vi "BRig_RT__Case_Exp__State_initBlock.vi"(0 "input_dataCurrent":u16[](array[numeric]), 3 "input_dataExp":u16[](array[numeric]), 4 "input_dataBlock":u16[][](array[numeric]), 5 "input_dataTrial":u16[][](array[numeric])) -> (6 "output_iSpout":u16, 7 "output_speaker_amp_R":u16, 8 "output_iBlock":u16, 9 "output_speaker_freq_R":u8, 10 "output_BUR_target":u16, 11 "output_speaker_amp_L":u16, 12 "output_TpB_target":u16, 13 "output_speaker_freq_L":u8, 14 "output_dataCurrent":u16[](array[numeric]), 18 "output_dataBlock":u16[][](array[numeric]), 19 "output_dataTrial":u16[][](array[numeric]))   [LabVIEW 2014]
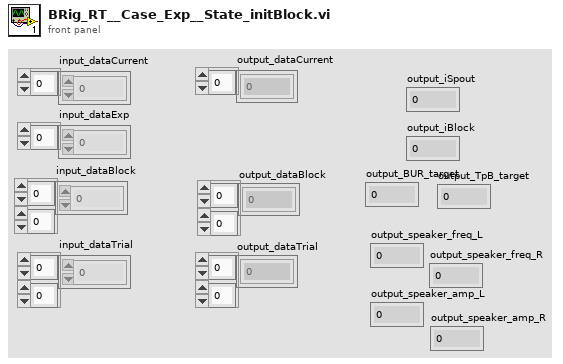
[diagram p1: front panel]
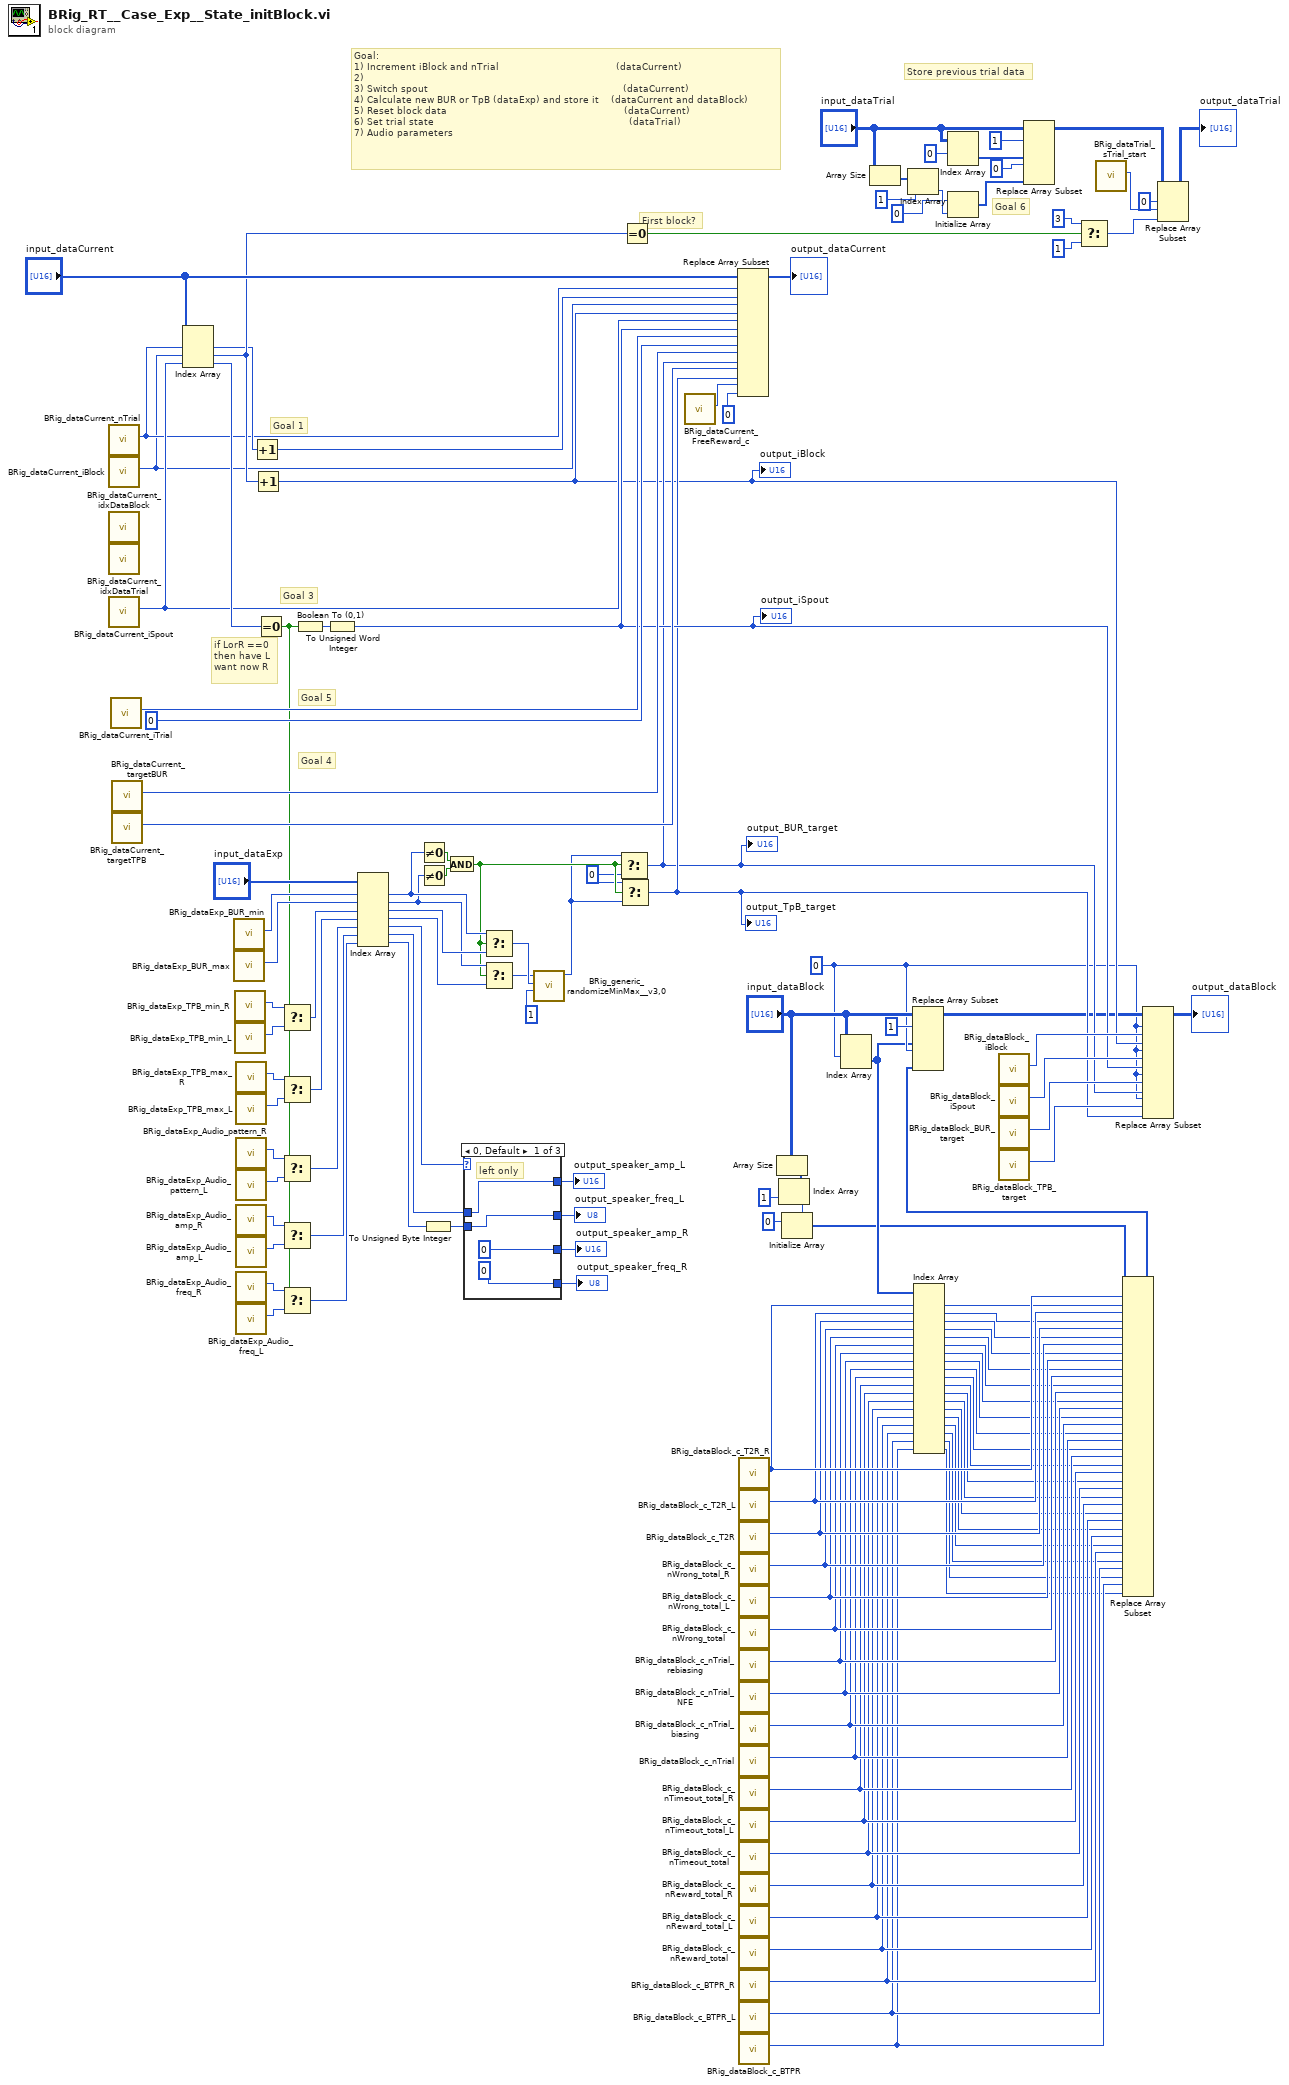
[diagram p0: block diagram]
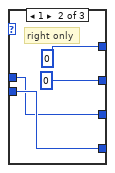
[diagram p2: hidden frame]
diagram:
  w43 = 0 ("disabled index (row)")
  w110 = u16 0 ("f")
  # "Store previous trial data"
  # "if LorR ==0\nthen have L\nwant now R"
  # "First block?"
  # "Goal 6"
  # "Goal 4"
  # "Goal 5"
  # "Goal 3"
  # "Goal 1"
  # "Goal:\n1) Increment iBlock and nTrial                                       (dataCurrent)\n2) \n3) Switch spout                                                                 (dataCurrent)\n4) Calculate new BUR or TpB (dataExp) and store it    (dataCurrent and dataBlock)\n5) Reset block data                                                           (dataCurrent)\n6) Set trial state                                                                 (dataTrial)\n7) Audio parameters"
  n1 = call "BRig_dataCurrent_nTrial.vi"() -> ("output_nTrial"=w65:i32)  [unwired: 11 in]
  n2 = call "BRig_dataCurrent_iBlock.vi"() -> ("output_iBlock"=w63:i32)  [unwired: 11 in]
  n3 = call "BRig_dataCurrent_idxDataBlock.vi"() -> ()  [unwired: 11 in, 1 out]
  n4 = call "BRig_dataCurrent_idxDataTrial.vi"() -> ()  [unwired: 11 in, 1 out]
  n5 = call "BRig_dataCurrent_iSpout.vi"() -> ("output_iSpout"=w93:i32)  [unwired: 11 in]
  n6 = call "BRig_dataCurrent_iTrial.vi"() -> ("output_iTrial"=w95:i32)  [unwired: 11 in]
  n7 = call "BRig_dataCurrent_targetBUR.vi"() -> ("output_targetBUR"=w97:i32)  [unwired: 11 in]
  n8 = call "BRig_dataCurrent_targetTPB.vi"() -> ("output_targetTPB"=w98:i32)  [unwired: 11 in]
  n9 = Index Array(array="input_dataCurrent", index #1=w65, index #2=w63, index #3=w93) -> (element #1=w92:u16, element #2=w104:u16, element #3=w129:u16)
  n10 = call "BRig_dataExp_BUR_min.vi"() -> ("output_BUR_min"=w127:i32)  [unwired: 11 in]
  n11 = call "BRig_dataExp_BUR_max.vi"() -> ("output_BUR_max"=w126:i32)  [unwired: 11 in]
  n12 = call "BRig_dataExp_TPB_min_R.vi"() -> ("output_TPB_min_R"=w122:i32)  [unwired: 11 in]
  n13 = call "BRig_dataExp_TPB_min_L.vi"() -> ("output_TPB_min_L"=w121:i32)  [unwired: 11 in]
  n14 = call "BRig_dataExp_TPB_max_R.vi"() -> ("output_TPB_max_R"=w68:i32)  [unwired: 11 in]
  n15 = call "BRig_dataExp_TPB_max_L.vi"() -> ("output_TPB_max_L"=w67:i32)  [unwired: 11 in]
  n16 = call "BRig_dataExp_Audio_pattern_R.vi"() -> ("output_Audio_sp__R"=w90:i32)  [unwired: 11 in]
  n17 = call "BRig_dataExp_Audio_pattern_L.vi"() -> ("output_Audio_sp__L"=w89:i32)  [unwired: 11 in]
  n18 = call "BRig_dataExp_Audio_amp_R.vi"() -> ("output_Audio_amp__R"=w88:i32)  [unwired: 11 in]
  n19 = call "BRig_dataExp_Audio_amp_L.vi"() -> ("output_Audio_amp__L"=w87:i32)  [unwired: 11 in]
  n20 = call "BRig_dataExp_Audio_freq_R.vi"() -> ("output_Audio_freq__R"=w86:i32)  [unwired: 11 in]
  n21 = call "BRig_dataExp_Audio_freq_L.vi"() -> ("output_Audio_freq__L"=w85:i32)  [unwired: 11 in]
  n22 = Increment(x=w92) -> (x+1=w64:u16)
  n23 = Increment(x=w104) -> (x+1=w62:u16)
  "output_iBlock" <- w62
  n24 = Equal To 0?(x=w129) -> (x = 0?=w91:bool)
  n25 = Select(t=w122, s=w91, f=w121) -> (s? t:f=w120:i32)
  n26 = Select(t=w68, s=w91, f=w67) -> (s? t:f=w119:i32)
  n27 = Select(t=w90, s=w91, f=w89) -> (s? t:f=w84:i32)
  n28 = Select(t=w88, s=w91, f=w87) -> (s? t:f=w83:i32)
  n29 = Select(t=w86, s=w91, f=w85) -> (s? t:f=w82:i32)
  n30 = Boolean To (0,1)(Boolean=w91) -> (0, 1=w130:i16)
  n31 = To Unsigned Word Integer(number=w130) -> (unsigned 16bit integer=w94:u16)
  "output_iSpout" <- w94
  n32 = Index Array(array="input_dataExp", index #1=w127, index #2=w126, index #3=w120, index #4=w119, index #5=w84, index #6=w83, index #7=w82) -> (element #1=w118:u16, element #2=w116:u16, element #3=w117:u16, element #4=w115:u16, element #5=w81:u16, element #6=w80:u16, element #7=w79:u16)
  n33 = Not Equal To 0?(x=w118) -> (x != 0?=w124:bool)
  n34 = Not Equal To 0?(x=w116) -> (x != 0?=w125:bool)
  n35 = To Unsigned Byte Integer(number=w79) -> (unsigned 8bit integer=w78:u8)
  n36 = And(x=w124, y=w125) -> (x .and. y?=w111:bool)
  n37 = case shown="0, Default" w81 {
    tunnel: w80 -> [w135 w138 w140]
    tunnel: w78 -> [w134 w139 w141]
    tunnel: [w135 u16 0 ("Numeric") w140] -> w77
    tunnel: [w134 u8 0 w141] -> w76
    tunnel: [u8 0 w139 w141] -> w75
    tunnel: [u16 0 ("Numeric") w138 w140] -> w74
    frame 0, Default {
      # "left only"
    }
    frame 1 {
      # "right only"
    }
    frame 2 {
      # "left and right"
    }
  }
  "output_speaker_amp_L" <- w77
  "output_speaker_freq_L" <- w76
  "output_speaker_amp_R" <- w74
  "output_speaker_freq_R" <- w75
  n38 = Select(t=w118, s=w111, f=w117) -> (s? t:f=w113:u16)
  n39 = Select(t=w116, s=w111, f=w115) -> (s? t:f=w112:u16)
  n40 = call "BRig_generic_randomizeMinMax__v3,0.vi"("Input_Increment"=u16 1, "Input_Min"=w113, "Input_Max"=w112) -> ("Output"=w109:u16)  [unwired: 8 in]
  n41 = Select(t=w109, s=w111, f=w110) -> (s? t:f=w72:u16)
  "output_BUR_target" <- w72
  n42 = Select(t=w110, s=w111, f=w109) -> (s? t:f=w73:u16)
  "output_TpB_target" <- w73
  n43 = Equal To 0?(x=w104) -> (x = 0?=w71:bool)
  n44 = call "BRig_dataCurrent_FreeReward_c.vi"() -> ("output_FreeReward_c"=w70:i32)  [unwired: 11 in]
  n45 = Replace Array Subset(array="input_dataCurrent", new element #1=w64, index #1=w65, new element #2=w62, index #2=w63, new element #3=w94, index #3=w93, new element #4=u16 0 ("new element/subarray"), index #4=w95, new element #5=w72, index #5=w97, new element #6=w73, index #6=w98, new element #7=u16 0 ("new element/subarray"), index #7=w70) -> (→"output_dataCurrent":u16[])
  n46 = call "BRig_dataBlock_c_T2R_R.vi"() -> ("output_c_T2R_R"=w38:i32)  [unwired: 11 in]
  n47 = call "BRig_dataBlock_c_T2R_L.vi"() -> ("output_c_T2R_L"=w37:i32)  [unwired: 11 in]
  n48 = call "BRig_dataBlock_c_T2R.vi"() -> ("output_c_T2R"=w36:i32)  [unwired: 11 in]
  n49 = call "BRig_dataBlock_c_nWrong_total_R.vi"() -> ("output_c_nWrong_total_R"=w35:i32)  [unwired: 11 in]
  n50 = call "BRig_dataBlock_c_nWrong_total_L.vi"() -> ("output_c_nWrong_total_L"=w34:i32)  [unwired: 11 in]
  n51 = call "BRig_dataBlock_c_nWrong_total.vi"() -> ("output_c_nWrong_total"=w33:i32)  [unwired: 11 in]
  n52 = call "BRig_dataBlock_c_nTrial_rebiasing.vi"() -> ("output_c_nTrial_rebiasing"=w32:i32)  [unwired: 11 in]
  n53 = call "BRig_dataBlock_c_nTrial_NFE.vi"() -> ("output_c_nTrial_NFE"=w31:i32)  [unwired: 11 in]
  n54 = call "BRig_dataBlock_c_nTrial_biasing.vi"() -> ("output_c_nTrial_biasing"=w30:i32)  [unwired: 11 in]
  n55 = call "BRig_dataBlock_c_nTrial.vi"() -> ("output_c_nTrial"=w29:i32)  [unwired: 11 in]
  n56 = call "BRig_dataBlock_c_nTimeout_total_R.vi"() -> ("output_c_nTimeout_total_R"=w28:i32)  [unwired: 11 in]
  n57 = call "BRig_dataBlock_c_nTimeout_total_L.vi"() -> ("output_c_nTimeout_total_L"=w27:i32)  [unwired: 11 in]
  n58 = call "BRig_dataBlock_c_nTimeout_total.vi"() -> ("output_c_nTimeout_total"=w26:i32)  [unwired: 11 in]
  n59 = call "BRig_dataBlock_c_nReward_total_R.vi"() -> ("output_nReward_total_R"=w25:i32)  [unwired: 11 in]
  n60 = call "BRig_dataBlock_c_nReward_total_L.vi"() -> ("output_nReward_total_L"=w24:i32)  [unwired: 11 in]
  n61 = call "BRig_dataBlock_c_nReward_total.vi"() -> ("output_nReward_total"=w23:i32)  [unwired: 11 in]
  n62 = call "BRig_dataBlock_c_BTPR_R.vi"() -> ("output_c_BTPR_R"=w22:i32)  [unwired: 11 in]
  n63 = call "BRig_dataBlock_c_BTPR_L.vi"() -> ("output_c_BTPR_L"=w21:i32)  [unwired: 11 in]
  n64 = call "BRig_dataBlock_c_BTPR.vi"() -> ("output_c_BTPR"=w20:i32)  [unwired: 11 in]
  n65 = Array Size(array="input_dataBlock") -> (size(s)=w50:i32[])
  n66 = Index Array(array=w50, index=1) -> (element=w48:i32)
  n67 = Initialize Array(u16 0 ("index"), w48) -> (w40:u16[])
  n68 = Index Array(array="input_dataBlock", index (row)=w43) -> (element=w41:u16[])  [unwired: 1 in]
  n69 = Array Size(array="input_dataTrial") -> (size(s)=w56:i32[])
  n70 = Index Array(array=w56, index=1) -> (element=w54:i32)
  n71 = Index Array(array=w41, index #1=w38, index #2=w37, index #3=w36, index #4=w35, index #5=w34, index #6=w33, index #7=w32, index #8=w31, index #9=w30, index #10=w29, index #11=w28, index #12=w27, index #13=w26, index #14=w25, index #15=w24, index #16=w23, index #17=w22, index #18=w21, index #19=w20) -> (element #1=w1:u16, element #2=w2:u16, element #3=w3:u16, element #4=w4:u16, element #5=w5:u16, element #6=w6:u16, element #7=w7:u16, element #8=w8:u16, element #9=w9:u16, element #10=w10:u16, element #11=w11:u16, element #12=w12:u16, element #13=w13:u16, element #14=w14:u16, element #15=w15:u16, element #16=w16:u16, element #17=w17:u16, element #18=w18:u16, element #19=w19:u16)
  n72 = Index Array(array="input_dataTrial", index (row)=0) -> (element=w58:u16[])  [unwired: 1 in]
  n73 = Initialize Array(u16 0 ("index"), w54) -> (w51:u16[])
  n74 = call "BRig_dataBlock_iBlock.vi"() -> ("output_iBlock"=w108:i32)  [unwired: 11 in]
  n75 = call "BRig_dataBlock_iSpout.vi"() -> ("output_iSpout"=w107:i32)  [unwired: 11 in]
  n76 = call "BRig_dataBlock_BUR_target.vi"() -> ("output_BUR_target"=w106:i32)  [unwired: 11 in]
  n77 = call "BRig_dataBlock_TPB_target.vi"() -> ("output_TPB_target"=w105:i32)  [unwired: 11 in]
  n78 = Replace Array Subset(array="input_dataTrial", new element #1=w58, index (row) #1=1 ("index (row)"), new element #2=w51, index (row) #2=0 ("index (row)")) -> (w61:u16[][])  [unwired: 2 in]
  n79 = Select(t=u16 3 ("new element/subarray"), s=w71, f=u16 1 ("new element/subarray")) -> (s? t:f=w102:u16)
  n80 = call "BRig_dataTrial_sTrial_start.vi"() -> ("output_sTrial_start"=w103:i32)  [unwired: 11 in]
  n81 = Replace Array Subset(array=w40, new element #1=w1, index #1=w38, new element #2=w2, index #2=w37, new element #3=w3, index #3=w36, new element #4=w4, index #4=w35, new element #5=w5, index #5=w34, new element #6=w6, index #6=w33, new element #7=w7, index #7=w32, new element #8=w8, index #8=w31, new element #9=w9, index #9=w30, new element #10=w10, index #10=w29, new element #11=w11, index #11=w28, new element #12=w12, index #12=w27, new element #13=w13, index #13=w26, new element #14=w14, index #14=w25, new element #15=w15, index #15=w24, new element #16=w16, index #16=w23, new element #17=w17, index #17=w22, new element #18=w18, index #18=w21, new element #19=w19, index #19=w20) -> (w39:u16[])
  n82 = Replace Array Subset(array="input_dataBlock", new element #1=w41, index (row) #1=1 ("index (row)"), new element #2=w39, index (row) #2=w43) -> (w44:u16[][])  [unwired: 2 in]
  n83 = Replace Array Subset(array=w44, new element #1=w62, index (row) #1=w43, index (col) #1=w108, new element #2=w94, index (row) #2=w43, index (col) #2=w107, new element #3=w72, index (row) #3=w43, index (col) #3=w106, new element #4=w73, index (row) #4=w43, index (col) #4=w105) -> (→"output_dataBlock":u16[][])
  n84 = Replace Array Subset(array=w61, new element=w102, index (row)=0 ("disabled index (row)"), index (col)=w103) -> (→"output_dataTrial":u16[][])
